vi "ZUP Write Single Message.vi"(8 "error in (no error)":errorcluster, 9 "Read Response":bool, 10 "Command Out":string, 11 "VISA resource name":refnum<visa-resource-name>) -> (0 "error out":errorcluster, 1 "Serial Settings:Number of Bytes at Serial Port":u32, 2 "Received Message":string, 3 "VISA OUT":refnum<visa-resource-name>)   [LabVIEW 2018]
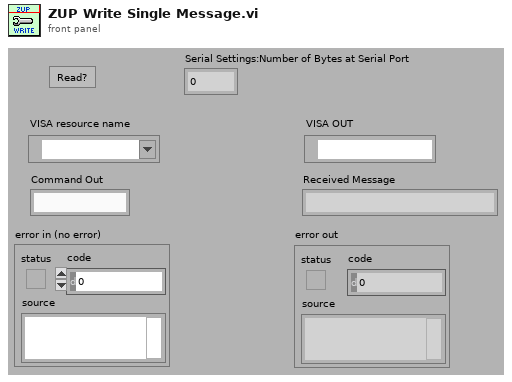
[diagram p1: front panel]
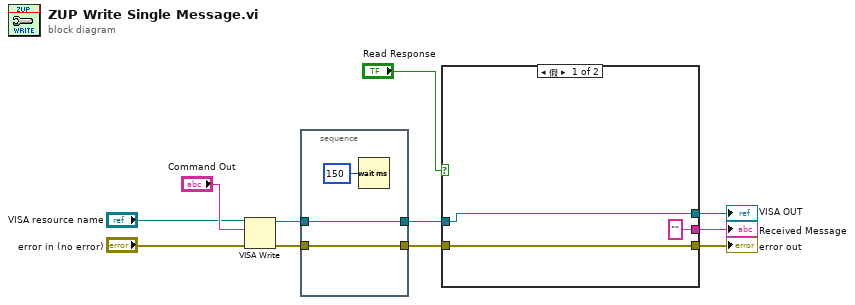
[diagram p0: block diagram]
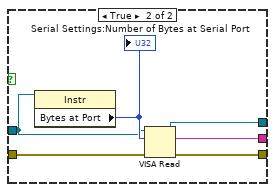
[diagram p2: hidden frame]
diagram:
  n1 = VISA Write(VISA resource name="VISA resource name", write buffer="Command Out", error in (no error)="error in (no error)") -> (VISA resource name out=w10:refnum<visa-resource-name>, error out=w11:errorcluster)  [unwired: 1 out]
  n2 = stacked-sequence {
    tunnel: w10 -> [w13]
    tunnel: [w13] -> w4
    tunnel: w11 -> [w12]
    tunnel: [w12] -> w5
    frame #0 {
      n3 = Wait (ms)(milliseconds to wait=u32 150) -> ()  [unwired: 1 out]
    }
  }
  n4 = case shown="假" "Read Response" {
    tunnel: [w16 w22] -> w9
    tunnel: [w17 w21] -> w1
    tunnel: ["" ("read buffer") w20] -> w7
    tunnel: w5 -> [w16 w19]
    tunnel: w4 -> [w17 w18]
    frame False {
    }
    frame True {
      n5 = property class="Instr"(reference=w18) -> ("Bytes at Port"=w23:u32)  [unwired: 1 in, 2 out]
      "Serial Settings:Number of Bytes at Serial Port" <- w23
      n6 = VISA Read(VISA resource name=w18, byte count=w23, error in (no error)=w19) -> (VISA resource name out=w21:refnum<visa-resource-name>, read buffer=w20:string, error out=w22:errorcluster)  [unwired: 1 out]
    }
  }
  "error out" <- w9
  "Received Message" <- w7
  "VISA OUT" <- w1
